vi "Rectangel LineIntersectLine.vi"(0 "LineA-Point1(l1p1)":T1 {"y" format="%.2f"; "x" format="%.2f"}, 1 "LineA-Point2(l1p2)":T1 {"y" format="%.2f"; "x" format="%.2f"}, 3 "LineB-Point1(l2p1)":T1 {"y" format="%.2f"; "x" format="%.2f"}, 4 "LineB-Point2(l2p2)":T1 {"y" format="%.2f"; "x" format="%.2f"}, 5 "error in (no error)":errorcluster) -> (15 "Intersect":bool, 19 "error out":errorcluster)   [LabVIEW 2020]
doc: "contains"
uses:
  <resource>/Framework/Providers/Open_GDS/UML/General/Point/Point Point2D.ctl
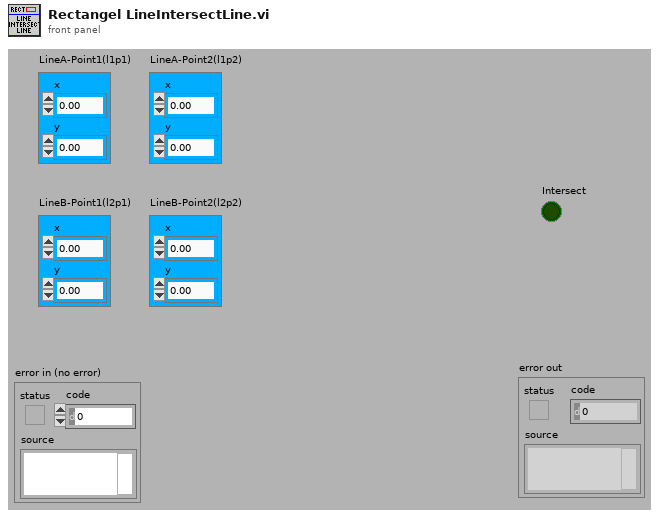
[diagram p1: front panel]
types:
  T1 = typedef "Point Point2D.ctl" = cluster{"x":dbl, "y":dbl}
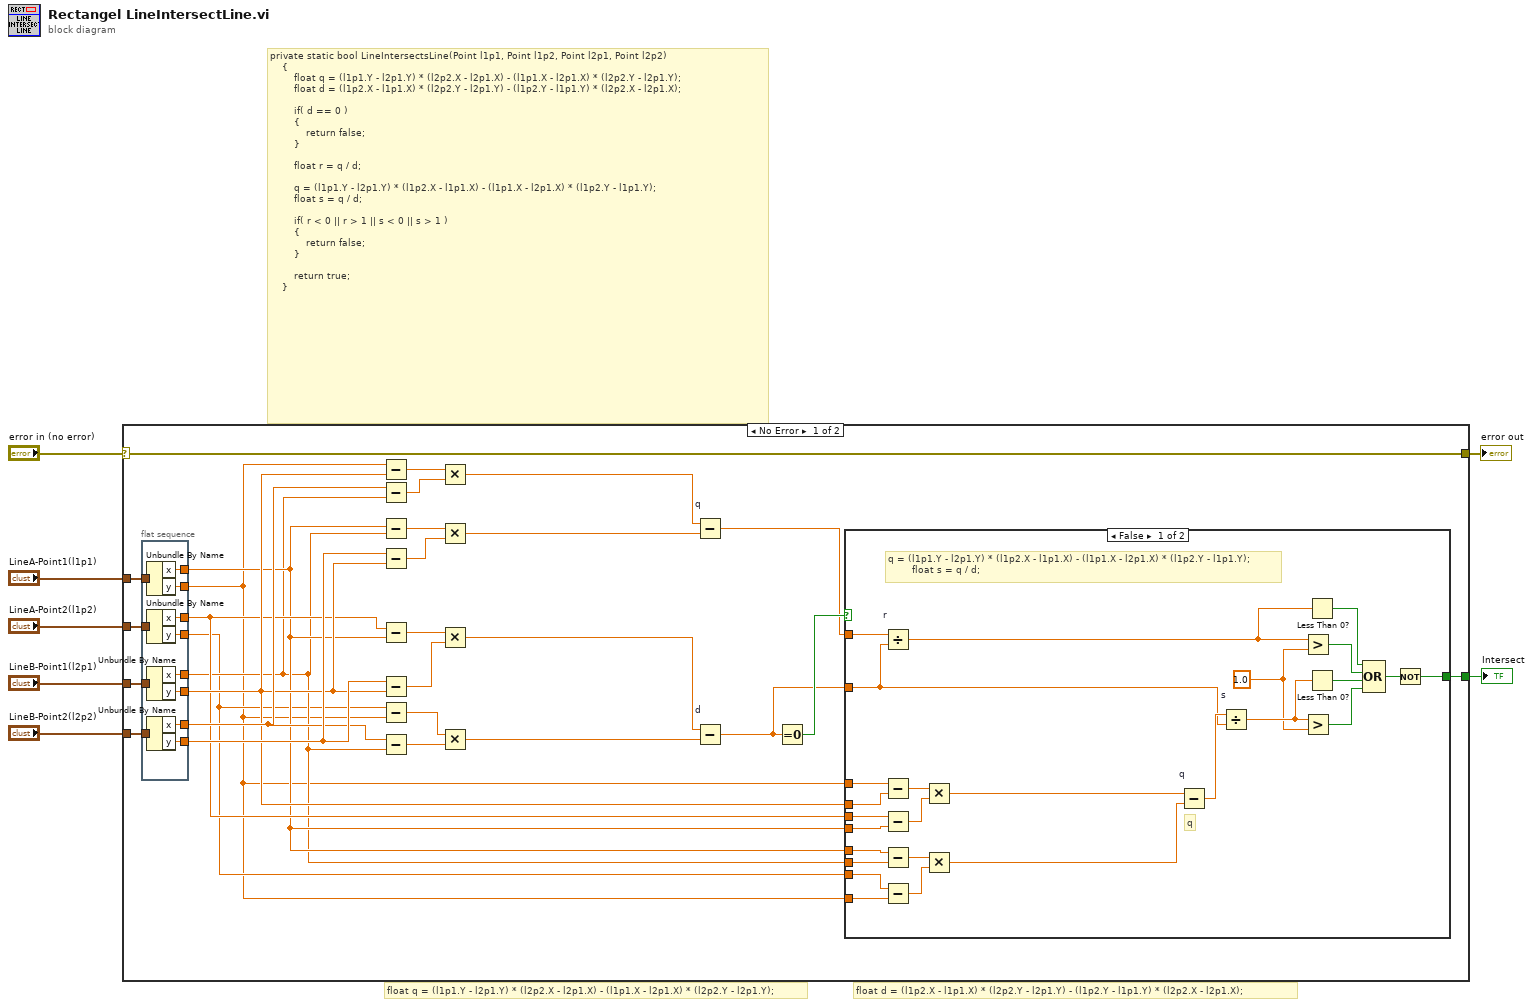
[diagram p0: block diagram]
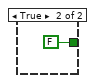
[diagram p2: hidden frame]
diagram:
  # "float q = (l1p1.Y - l2p1.Y) * (l2p2.X - l2p1.X) - (l1p1.X - l2p1.X) * (l2p2.Y - l2p1.Y);"
  # "float d = (l1p2.X - l1p1.X) * (l2p2.Y - l2p1.Y) - (l1p2.Y - l1p1.Y) * (l2p2.X - l2p1.X);"
  # "private static bool LineIntersectsLine(Point l1p1, Point l1p2, Point l2p1, Point l2p2)\n    {\n        float q = (l1p1.Y - l2p1.Y) * (l2p2.X - l2p1.X) - (l1p1.X - l2p1.X) * (l2p2.Y - l2p1.Y);\n        float d = (l1p2.X - l1p1.X) * (l2p2.Y - l2p1.Y) - (l1p2.Y - l1p1.Y) * (l2p2.X - l2p1.X);\n\n        if( d == 0 )\n        {\n            return false;\n        }\n\n        float r = q / d;\n\n        q = (l1p1.Y - l2p1.Y) * (l1p2.X - l1p1.X) - (l1p1.X - l2p1.X) * (l1p2.Y - l1p1.Y);\n        float s = q / d;\n\n        if( r < 0 || r > 1 || s < 0 || s > 1 )\n        {\n            return false;\n        }\n\n        return true;\n    }"
  n1 = case shown="No Error" "error in (no error)" {
    selector: "error in (no error)" -> [w36 w76]
    tunnel: [w36 w76] -> w7
    tunnel: "LineA-Point1(l1p1)" -> [w35 _]
    tunnel: "LineA-Point2(l1p2)" -> [w34 _]
    tunnel: "LineB-Point2(l2p2)" -> [w32 _]
    tunnel: "LineB-Point1(l2p1)" -> [w33 _]
    tunnel: [w18 _] -> w1
    frame No Error {
      n2 = flat-sequence {
        tunnel: w35 -> [w48]
        tunnel: w34 -> [w47]
        tunnel: w33 -> [w46]
        tunnel: w32 -> [w45]
        tunnel: [w44] -> w12
        tunnel: [w43] -> w11
        tunnel: [w42] -> w15
        tunnel: [w41] -> w13
        tunnel: [w40] -> w8
        tunnel: [w39] -> w14
        tunnel: [w38] -> w10
        tunnel: [w37] -> w9
        frame #0 {
          n3 = Unbundle By Name(w48) -> ("x"=w43:dbl, "y"=w40:dbl)
          n4 = Unbundle By Name(w47) -> ("x"=w44:dbl, "y"=w37:dbl)
          n5 = Unbundle By Name(w46) -> ("x"=w38:dbl, "y"=w41:dbl)
          n6 = Unbundle By Name(w45) -> ("x"=w39:dbl, "y"=w42:dbl)
        }
      }
      n7 = Subtract(x=w8, y=w13) -> (x-y=w29:dbl)
      n8 = Subtract(x=w14, y=w10) -> (x-y=w30:dbl)
      n9 = Subtract(x=w11, y=w10) -> (x-y=w31:dbl)
      n10 = Subtract(x=w15, y=w13) -> (x-y=w20:dbl)
      n11 = Subtract(x=w12, y=w11) -> (x-y=w24:dbl)
      n12 = Subtract(x=w15, y=w13) -> (x-y=w23:dbl)
      n13 = Subtract(x=w9, y=w8) -> (x-y=w21:dbl)
      n14 = Subtract(x=w14, y=w10) -> (x-y=w22:dbl)
      n15 = Multiply(x=w29, y=w30) -> (x*y=w28:dbl)
      n16 = Multiply(x=w31, y=w20) -> (x*y=w27:dbl)
      n17 = Multiply(x=w24, y=w23) -> (x*y=w25:dbl)
      n18 = Multiply(x=w21, y=w22) -> (x*y=w26:dbl)
      n19 = Subtract "q"(x=w28, y=w27) -> (x-y=w17:dbl)
      n20 = Subtract "d"(x=w25, y=w26) -> (x-y=w16:dbl)
      n21 = Equal To 0?(x=w16) -> (x = 0?=w19:bool)
      n22 = case shown="False" w19 {
        tunnel: [w49 FALSE] -> w18
        tunnel: w17 -> [w74 _]
        tunnel: w16 -> [w58 _]
        tunnel: w8 -> [w73 _]
        tunnel: w13 -> [w72 _]
        tunnel: w12 -> [w65 _]
        tunnel: w11 -> [w64 _]
        tunnel: w11 -> [w63 _]
        tunnel: w10 -> [w62 _]
        tunnel: w9 -> [w61 _]
        tunnel: w8 -> [w60 _]
        frame False {
          w55 = 1.0 ("y")
          # "q"
          # "q = (l1p1.Y - l2p1.Y) * (l1p2.X - l1p1.X) - (l1p1.X - l2p1.X) * (l1p2.Y - l1p1.Y);\n        float s = q / d;"
          n23 = Divide "r"(x=w74, y=w58) -> (x/y=w57:dbl)
          n24 = Subtract(x=w73, y=w72) -> (x-y=w71:dbl)
          n25 = Subtract(x=w65, y=w64) -> (x-y=w70:dbl)
          n26 = Subtract(x=w63, y=w62) -> (x-y=w68:dbl)
          n27 = Subtract(x=w61, y=w60) -> (x-y=w69:dbl)
          n28 = Multiply(x=w71, y=w70) -> (x*y=w67:dbl)
          n29 = Multiply(x=w68, y=w69) -> (x*y=w66:dbl)
          n30 = Subtract "q"(x=w67, y=w66) -> (x-y=w59:dbl)
          n31 = Divide "s"(x=w59, y=w58) -> (x/y=w56:dbl)
          n32 = Greater?(x=w57, y=w55) -> (0:w53:bool)
          n33 = Greater?(x=w56, y=w55) -> (0:w51:bool)
          n34 = Less Than 0?(x=w57) -> (x < 0?=w54:bool)
          n35 = Less Than 0?(x=w56) -> (x < 0?=w52:bool)
          n36 = Compound Arithmetic op=OR(w54, w53, w52, w51) -> (w50:bool)
          n37 = Not(x=w50) -> (.not. x?=w49:bool)
        }
        frame True {
        }
      }
    }
    frame Error {
    }
  }
  "error out" <- w7
  "Intersect" <- w1
